vi "Lab1_5.vi"() -> ()   [LabVIEW 2021]
panel:
  out "Modified Cluster":T1
  out "Boolean 2":bool
  out "Numeric":dbl
  out "Small Cluster":cluster{"Boolean":bool, "Slide":dbl}
  in  "stop":bool
  in  "Cluster":T1 {"Slide" scale=0.0..10.0}
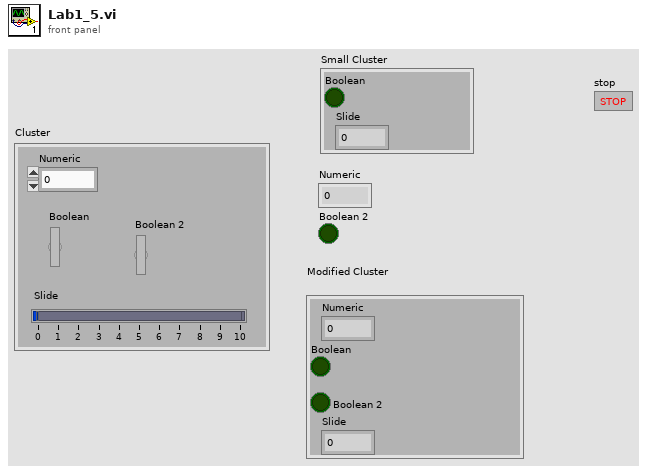
[diagram p1: front panel]
types:
  T1 = cluster{"Numeric":dbl, "Boolean":bool, "Boolean 2":bool, "Slide":dbl}
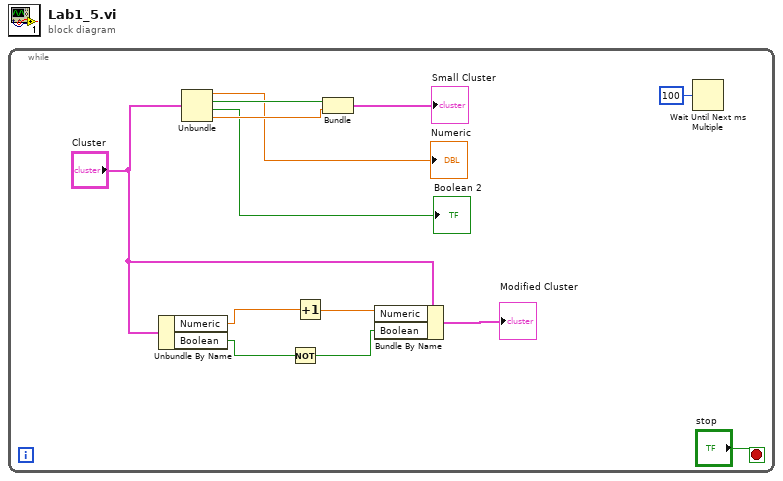
[diagram p0: block diagram]
diagram:
  n1 = while {
    stop <- "stop" stop-if-true
    n2 = Unbundle By Name "Unbundle By Name"("Cluster") -> ("Numeric"=w6:dbl, "Boolean"=w5:bool)
    n3 = Unbundle "Unbundle"("Cluster") -> ("Numeric"=→"Numeric":dbl, "Boolean"=w10:bool, "Boolean 2"=→"Boolean 2":bool, "Slide"=w11:dbl)
    n4 = Not(x=w5) -> (.not. x?=w2:bool)
    n5 = Increment(x=w6) -> (x+1=w3:dbl)
    n6 = Bundle("Boolean"=w10, "Slide"=w11) -> (→"Small Cluster":cluster{"Boolean":bool, "Slide":dbl})  [unwired: 1 in]
    n7 = Bundle By Name "Bundle By Name"(cluster="Cluster", "Numeric"=w3, "Boolean"=w2) -> (→"Modified Cluster":T1)
    n8 = Wait Until Next ms Multiple(millisecond multiple=u32 100) -> ()  [unwired: 1 out]
  }
